vi "Destroy.vi"(8 "error in (no error)":errorcluster, 11 "Group":refnum<class "Group.lvclass">) -> (0 "error out":errorcluster)   [LabVIEW 2021]
uses:
  Group.lvclass
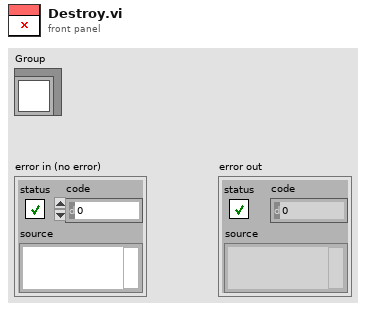
[diagram p1: front panel]
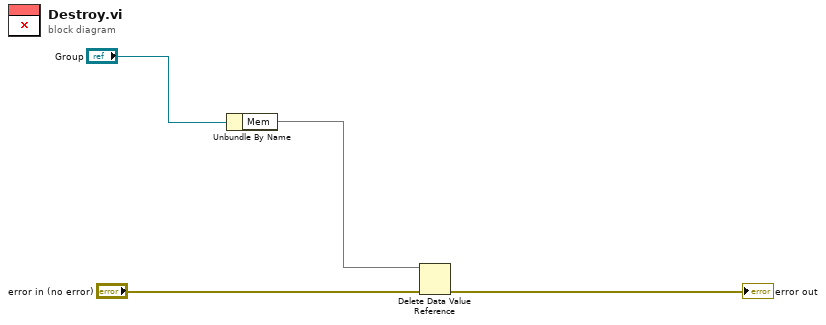
[diagram p0: block diagram]
diagram:
  n1 = Unbundle By Name("Group") -> ("Mem"=w1)
  n2 = Delete Data Value Reference(data value reference=w1, error in="error in (no error)") -> (error out=→"error out":errorcluster)  [unwired: 1 out]
